vi "Is File VI.vi"(8 "error in (no error)":errorcluster, 11 "path":path) -> (0 "error out":errorcluster, 2 "Is Class Private Data Control?":bool, 3 "Is VI?":bool)   [LabVIEW 2015, in "NI_FileType.lvlib"]
doc: "Returns TRUE if this file could be loaded with the Open VI Reference function. It includes VIs, Polymorphic VIs, Controls, Templates, and Globals."
uses:
  NI_FileType.lvlib
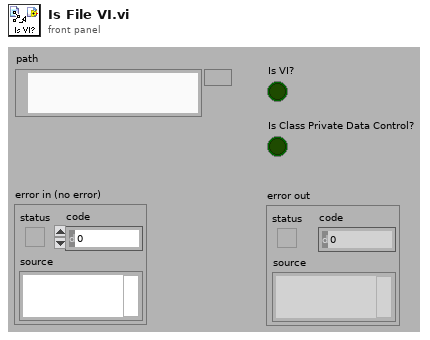
[diagram p1: front panel]
types:
  T1 = typedef "NI_FileType.lvlib/FT_FileTypes.ctl" = enum32{"Invalid file/path", "Unknown type", "Instrument", "Control", "Polymorphic VI", "Project", "Library", "LVClass", "XControl", "XNode", "CIN", "Run-time menu", "Palette menu", "LLB", "Shortcut", "Directory", "Class Private Data Control", "Statechart", "MathScript .m file", "Ladder Diagram", "LVLibp"}
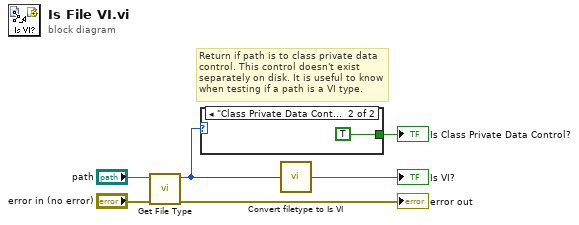
[diagram p0: block diagram]
diagram:
  # "Return if path is to class private data control. This control doesn't exist separately on disk. It is useful to know when testing if a path is a VI type."
  n1 = call "Get File Type.vi"("error in (no error)"="error in (no error)", "path"="path") -> ("error out"=→"error out":errorcluster, "file type"=w2:T1)  [unwired: 7 in, 1 out]
  n2 = case shown="\"Class Private Data Control\"" w2 {
    tunnel: [_ TRUE] -> w1
    frame Default {
    }
    frame "Class Private Data Control" {
    }
  }
  "Is Class Private Data Control?" <- w1
  n3 = call "Convert filetype to Is VI.vi"("file type"=w2) -> ("Is VI?"=→"Is VI?":bool)  [unwired: 4 in]
